vi "include.set.vi"(8 "error in (no error)":errorcluster, 10 "include":set{refnum<class "filterTypes.lvclass">}(c389), 11 "include in":refnum<class "include.lvclass">) -> (0 "error out":errorcluster, 3 "include out":refnum<class "include.lvclass">)   [LabVIEW 2020, in "nominal types.lvlib" / "channelFilter.lvlib" / "include.lvclass"]
uses:
  include.lvclass
  include.lvclass/include.ctl
  filterTypes/filterTypes.lvclass
  C:/code/labview-client/lv_src/nominal types/filterTypes/filterTypes.lvclass
  C:/code/labview-client/lv_src/Nominal Client/datasources/payload/payload.lvclass
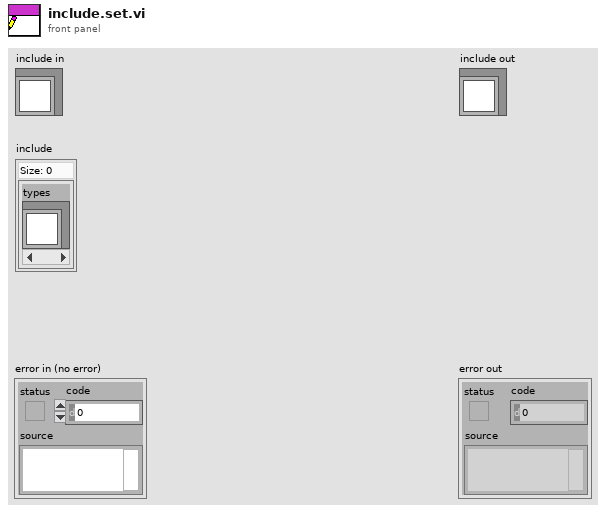
[diagram p1: front panel]
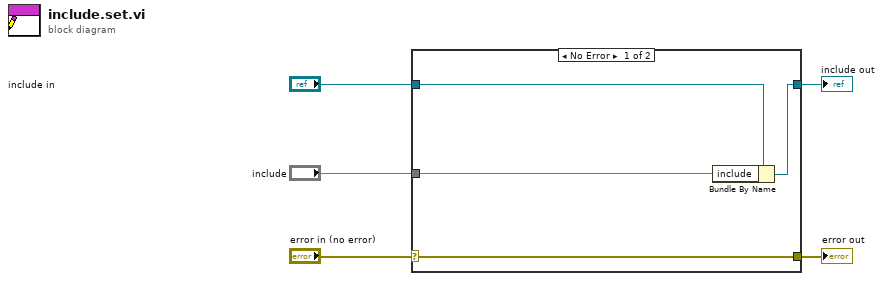
[diagram p0: block diagram]
diagram:
  n1 = case shown="No Error" "error in (no error)" {
    selector: "error in (no error)" -> [w9 w10]
    tunnel: [w9 w10] -> w4
    tunnel: [w7 w11] -> w2
    tunnel: "include in" -> [w8 w11]
    tunnel: "include" -> [w6 _]
    frame No Error {
      n2 = Bundle By Name(cluster=w8, "include"=w6) -> (w7:refnum<class "include.lvclass">)
    }
    frame Error {
    }
  }
  "error out" <- w4
  "include out" <- w2
